vi "Label PrintOut.vi"(6 "Model (F-ME74)":bool, 7 "Label Print Pass/Fail (F-Fail)":bool, 8 "error in (no error)":errorcluster, 9 "Fail Data":T1, 10 "Pass Data":T2, 11 "Labels Reference In":T3) -> (0 "error out":errorcluster)   [LabVIEW 2018]
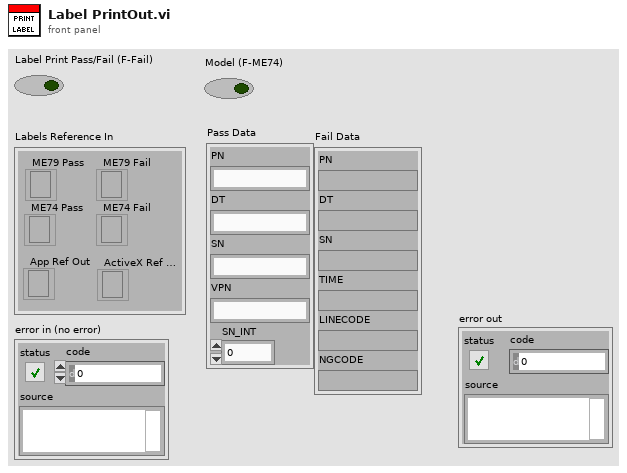
[diagram p1: front panel]
types:
  T1 = cluster{"PN":string, "DT":string, "SN":string, "TIME":string, "LINECODE":string, "NGCODE":string}
  T2 = cluster{"PN":string, "DT":string, "SN":string, "VPN":string, "SN_INT":i32}
  T3 = cluster{"ME79 Pass":refnum<k7>, "ME79 Fail":refnum<k7>, "ME74 Pass":refnum<k7>, "ME74 Fail":refnum<k7>, "App Ref Out":refnum<k7>, "ActiveX Ref Out":refnum<k7>}
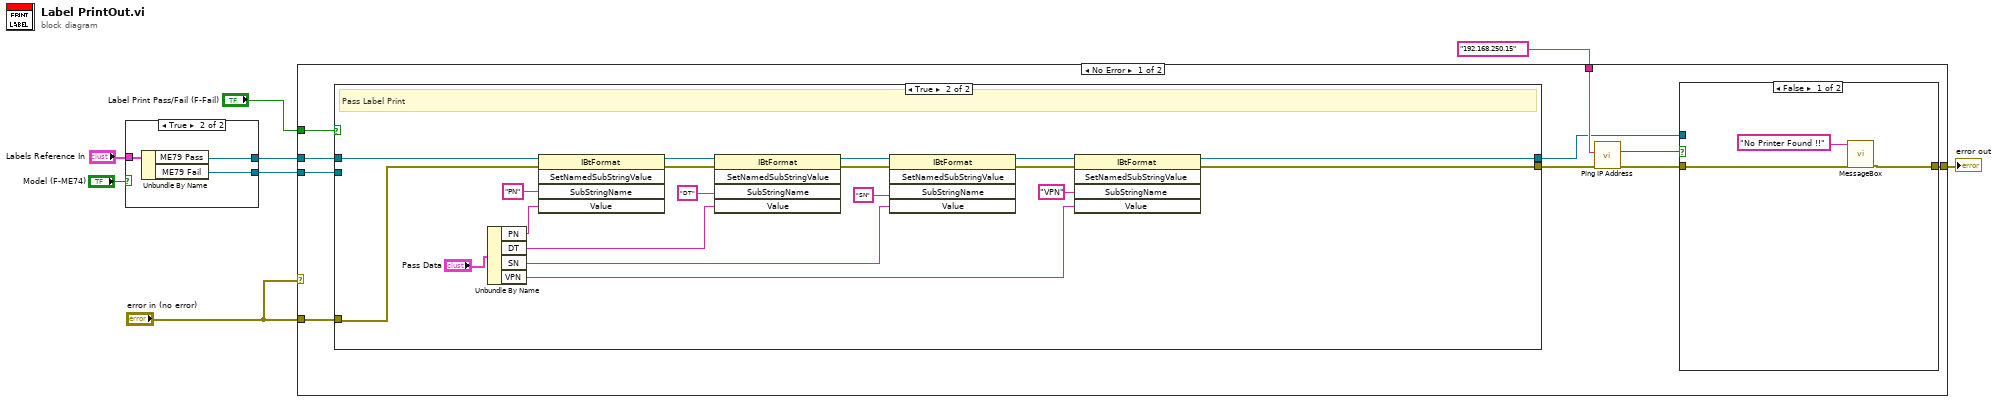
[diagram p0: block diagram]
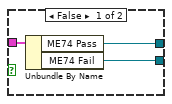
[diagram p2: hidden frame]
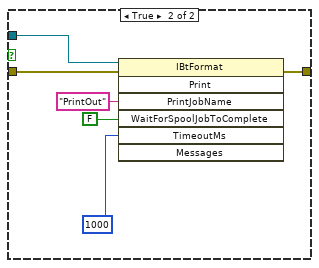
[diagram p3: hidden frame]
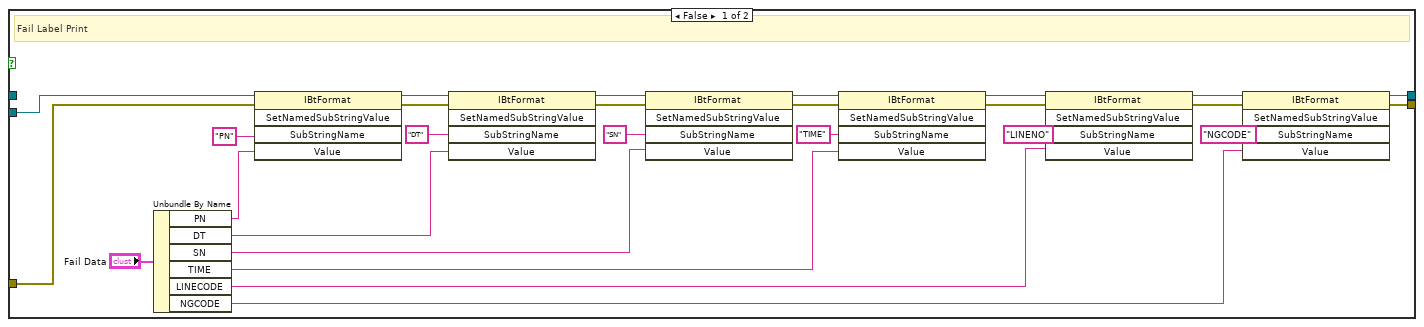
[diagram p4: hidden frame]
diagram:
  n1 = case shown="True" "Model (F-ME74)" {
    tunnel: "Labels Reference In" -> [w11 w14]
    tunnel: [w10 w13] -> w3
    tunnel: [w9 w12] -> w2
    frame False {
      n2 = Unbundle By Name(w11) -> ("ME74 Pass"=w10:refnum<k7>, "ME74 Fail"=w9:refnum<k7>)
    }
    frame True {
      n3 = Unbundle By Name(w14) -> ("ME79 Pass"=w13:refnum<k7>, "ME79 Fail"=w12:refnum<k7>)
    }
  }
  n4 = case shown="No Error" "error in (no error)" {
    tunnel: "error in (no error)" -> [w23 w80]
    tunnel: "Label Print Pass/Fail (F-Fail)" -> [w24 _]
    tunnel: w3 -> [w15 _]
    tunnel: [w22 w80] -> w7
    tunnel: w2 -> [w21 _]
    tunnel: "192.168.250.15" ("IP Address") -> [w19 _]
    frame No Error {
      n5 = case shown="True" w24 {
        tunnel: w23 -> [w35 w72]
        tunnel: [w42 w62] -> w20
        tunnel: w21 -> [w59 _]
        tunnel: [w34 w63] -> w16
        tunnel: w15 -> [_ w67]
        frame False {
          # "Fail Label Print"
          n6 = Unbundle By Name("Fail Data") -> ("PN"=w41:string, "DT"=w40:string, "SN"=w39:string, "TIME"=w38:string, "LINECODE"=w37:string, "NGCODE"=w36:string)
          n7 = invoke class="IBtFormat" method="SetNamedSubStringValue"(reference=w59, error in=w35, "SubStringName"="PN", "Value"=w41) -> (reference out=w52:refnum<k7>, error out=w48:errorcluster)  [unwired: 1 in, 3 out]
          n8 = invoke class="IBtFormat" method="SetNamedSubStringValue"(reference=w52, error in=w48, "SubStringName"="DT", "Value"=w40) -> (reference out=w51:refnum<k7>, error out=w47:errorcluster)  [unwired: 1 in, 3 out]
          n9 = invoke class="IBtFormat" method="SetNamedSubStringValue"(reference=w51, error in=w47, "SubStringName"="SN", "Value"=w39) -> (reference out=w50:refnum<k7>, error out=w46:errorcluster)  [unwired: 1 in, 3 out]
          n10 = invoke class="IBtFormat" method="SetNamedSubStringValue"(reference=w50, error in=w46, "SubStringName"="TIME", "Value"=w38) -> (reference out=w49:refnum<k7>, error out=w45:errorcluster)  [unwired: 1 in, 3 out]
          n11 = invoke class="IBtFormat" method="SetNamedSubStringValue"(reference=w49, error in=w45, "SubStringName"="LINENO", "Value"=w37) -> (reference out=w44:refnum<k7>, error out=w43:errorcluster)  [unwired: 1 in, 3 out]
          n12 = invoke class="IBtFormat" method="SetNamedSubStringValue"(reference=w44, error in=w43, "SubStringName"="NGCODE", "Value"=w36) -> (reference out=w34:refnum<k7>, error out=w42:errorcluster)  [unwired: 1 in, 3 out]
        }
        frame True {
          # "Pass Label Print"
          n13 = Unbundle By Name("Pass Data") -> ("PN"=w77:string, "DT"=w71:string, "SN"=w70:string, "VPN"=w61:string)
          n14 = invoke class="IBtFormat" method="SetNamedSubStringValue"(reference=w67, error in=w72, "SubStringName"="PN", "Value"=w77) -> (reference out=w73:refnum<k7>, error out=w69:errorcluster)  [unwired: 1 in, 3 out]
          n15 = invoke class="IBtFormat" method="SetNamedSubStringValue"(reference=w73, error in=w69, "SubStringName"="DT", "Value"=w71) -> (reference out=w74:refnum<k7>, error out=w68:errorcluster)  [unwired: 1 in, 3 out]
          n16 = invoke class="IBtFormat" method="SetNamedSubStringValue"(reference=w74, error in=w68, "SubStringName"="SN", "Value"=w70) -> (reference out=w65:refnum<k7>, error out=w64:errorcluster)  [unwired: 1 in, 3 out]
          n17 = invoke class="IBtFormat" method="SetNamedSubStringValue"(reference=w65, error in=w64, "SubStringName"="VPN", "Value"=w61) -> (reference out=w63:refnum<k7>, error out=w62:errorcluster)  [unwired: 1 in, 3 out]
        }
      }
      n18 = call "Ping IP Address.vi"("error in (no error)"=w20, "IP Address"=w19) -> ("error out"=w18:errorcluster, "Found?"=w17:bool)  [unwired: 8 in]
      n19 = case shown="False" w17 {
        tunnel: w16 -> [_ w33]
        tunnel: w18 -> [w27 w32]
        tunnel: [w26 w31] -> w22
        frame False {
          n20 = call "MessageBox.vi"("Error In"=w27, "Message"="No Printer Found !!" ("message")) -> ("Error Out"=w26:errorcluster)  [unwired: 9 in]
        }
        frame True {
          n21 = invoke class="IBtFormat" method="Print"(reference=w33, error in=w32, "PrintJobName"="PrintOut", "WaitForSpoolJobToComplete"=FALSE, "TimeoutMs"=1000) -> (error out=w31:errorcluster)  [unwired: 2 in, 6 out]
        }
      }
    }
    frame Error {
    }
  }
  "error out" <- w7
